vi "Update Monitor State.vi"(8 "error in (no error)":errorcluster, 10 "Monitor Running":bool, 11 "Monitor-Pulse in":refnum<class "Application Controller.lvclass">) -> (0 "error out":errorcluster, 3 "Monitor-Pulse out":refnum<class "Application Controller.lvclass">)   [LabVIEW 2016, in "Application Controller.lvclass"]
uses:
  Application Controller.lvclass
  Application Controller.lvclass/Application Controller.ctl
  Comms/Communications Messages/Set Topic Value Msg/Set Topic Value Msg.lvclass/Set Topic Value Msg.ctl
  <vilib>/ActorFramework/Message Enqueuer/Message Enqueuer.lvclass/Message Enqueuer.ctl
  Read Monitor Running.vi
  <vilib>/ActorFramework/Message Enqueuer/Enqueue.vi
  Comms/Communications Messages/Set Topic Value Msg/Set Topic Value Msg.lvclass
  C:/Program Files/National Instruments/LabVIEW 2016/vi.lib/ActorFramework/Message/Message.lvclass
  <vilib>/ActorFramework/Message Priority Queue/Priority Enqueue.vi
  <vilib>/ActorFramework/Message Enqueuer/Message Enqueuer.lvclass
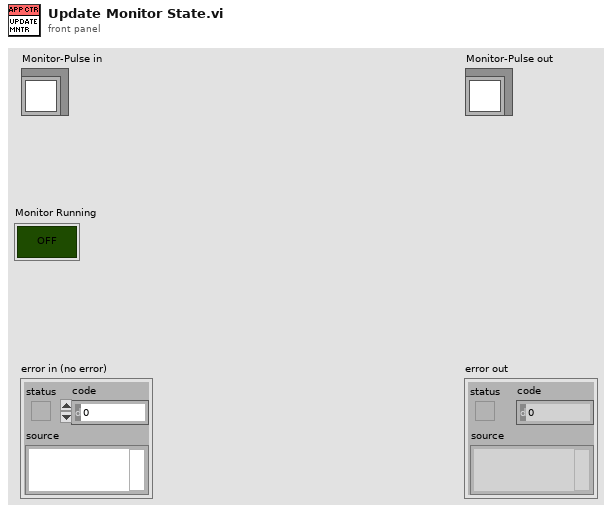
[diagram p1: front panel]
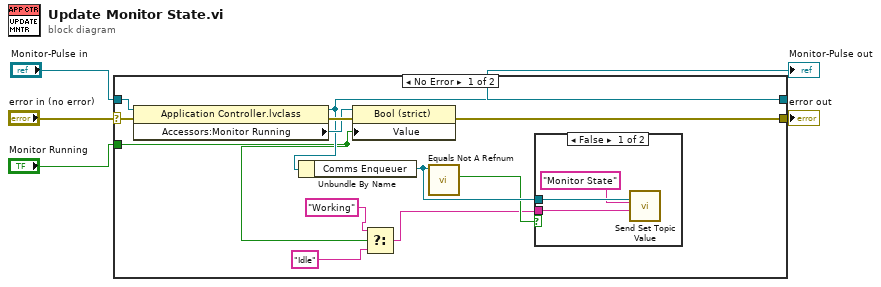
[diagram p0: block diagram]
diagram:
  n1 = case shown="No Error" "error in (no error)" {
    selector: "error in (no error)" -> [w17 w22]
    tunnel: [w16 w22] -> w4
    tunnel: [w10 w21] -> w2
    tunnel: "Monitor-Pulse in" -> [w14 w21]
    tunnel: "Monitor Running" -> [w9 _]
    frame No Error {
      n2 = property class="Application Controller.lvclass"(reference=w14, error in=w17) -> (reference out=w10:refnum<class "Application Controller.lvclass">, error out=w15:errorcluster, "Accessors:Monitor Running"=w13:refnum<vi>)
      n3 = Unbundle By Name(w10) -> ("Comms Enqueuer"=w12:refnum<class "Message Enqueuer.lvclass">)
      n4 = property class="Bool (strict)"(reference=w13, error in=w15, "Value"=w9) -> (error out=w16:errorcluster)  [unwired: 1 out]
      n5 = Select(t="Working", s=w9, f="Idle") -> (s? t:f=w6:string)
      n6 = call <vilib>:"Equals Not A Refnum.vi"("Message Enqueuer"=w12) -> ("Not a refnum?"=w11:bool)  [unwired: 10 in]
      n7 = case shown="False" w11 {
        tunnel: w12 -> [w20 _]
        tunnel: w6 -> [w19 _]
        frame False {
          n8 = call "Send Set Topic Value.vi"("Value"=w19, "Topic"="Monitor State", "Message Enqueuer"=w20) -> ()  [unwired: 7 in, 2 out]
        }
        frame True {
        }
      }
    }
    frame Error {
    }
  }
  "error out" <- w4
  "Monitor-Pulse out" <- w2
